vi "SubVI_EXA amplitude.vi"(5 "Enable Auto Attenuation (T: Enable)":bool, 6 "Manual Attenuation (30 dB)":dbl, 7 "Amplitude Units (0: dBm)":u16, 8 "error in (no error)":errorcluster, 9 "Reference Level Offset (0 dB)":dbl, 10 "Reference Level (0)":dbl, 11 "VISA Refnum in":refnum<visa-resource-name>) -> (0 "error out":errorcluster, 3 "VISA resource name":refnum<visa-resource-name>)   [LabVIEW 2016]
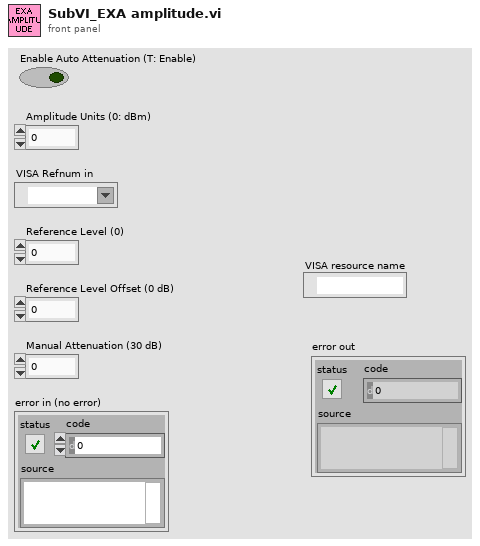
[diagram p1: front panel]
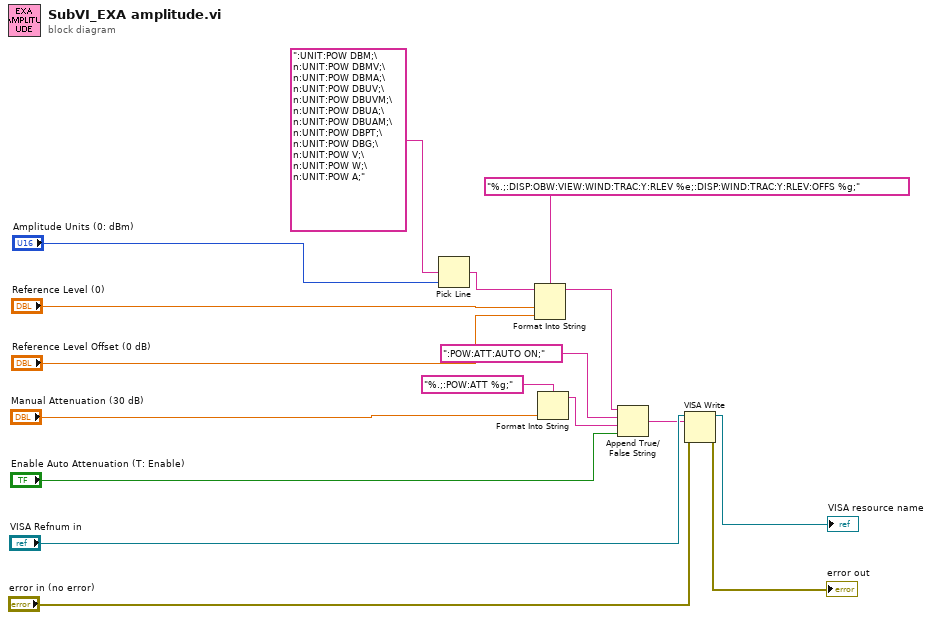
[diagram p0: block diagram]
diagram:
  n1 = Pick Line(multi-line string=":UNIT:POW DBM;\n:UNIT:POW DBMV;\n:UNIT:POW DBMA;\n:UNIT:POW DBUV;\n:UNIT:POW DBUVM;\n:UNIT:POW DBUA;\n:UNIT:POW DBUAM;\n:UNIT:POW DBPT;\n:UNIT:POW DBG;\n:UNIT:POW V;\n:UNIT:POW W;\n:UNIT:POW A;", line index="Amplitude Units (0: dBm)") -> (output string=w6:string)  [unwired: 1 in]
  n2 = Format Into String(format string="%.;:DISP:OBW:VIEW:WIND:TRAC:Y:RLEV %e;:DISP:WIND:TRAC:Y:RLEV:OFFS %g;", initial string=w6, "Reference Level (0)", "Reference Level Offset (0 dB)") -> (resulting string=w12:string)  [unwired: 1 in, 1 out]
  n3 = Format Into String(format string="%.;:POW:ATT %g;", "Manual Attenuation (30 dB)") -> (resulting string=w10:string)  [unwired: 2 in, 1 out]
  n4 = Append True/False String(1:"Enable Auto Attenuation (T: Enable)", 2:w10, 3:":POW:ATT:AUTO ON;" ("string (\"\")"), 4:w12) -> (0:w13:string)
  n5 = VISA Write(VISA resource name="VISA Refnum in", write buffer=w13, error in (no error)="error in (no error)") -> (VISA resource name out=→"VISA resource name":refnum<visa-resource-name>, error out=→"error out":errorcluster)  [unwired: 1 out]
